vi "Read TCPClient.vi"(8 "error in (no error)":errorcluster, 11 "SpectrographClientCommunicator in":refnum<class "SpectrographClientCommunicator.lvclass">) -> (0 "error out":errorcluster, 2 "TCPClient":refnum<class "TCPClient.lvclass">, 3 "SpectrographClientCommunicator out":refnum<class "SpectrographClientCommunicator.lvclass">)   [LabVIEW 2016, in "SpectrographClientCommunicator.lvclass"]
uses:
  SpectrographClientCommunicator.lvclass
  ts_labview_tcp/TCPClient/TCPClient.lvclass
  SpectrographClientCommunicator.lvclass/SpectrographClientCommunicator.ctl
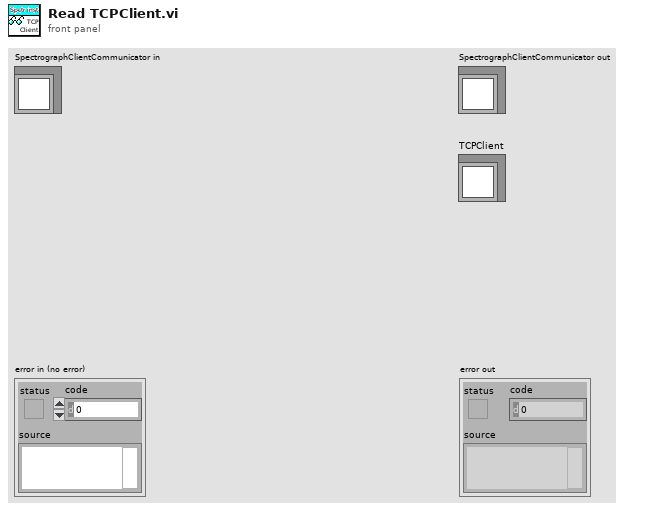
[diagram p1: front panel]
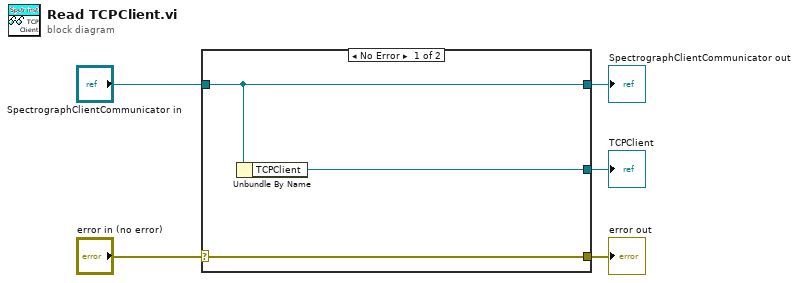
[diagram p0: block diagram]
diagram:
  n1 = case shown="No Error" "error in (no error)" {
    selector: "error in (no error)" -> [w8 w9]
    tunnel: [w8 w9] -> w4
    tunnel: [w7 w10] -> w2
    tunnel: "SpectrographClientCommunicator in" -> [w7 w10]
    tunnel: [w6 _] -> w1
    frame No Error {
      n2 = Unbundle By Name(w7) -> ("TCPClient"=w6:refnum<class "TCPClient.lvclass">)
    }
    frame Error {
    }
  }
  "error out" <- w4
  "SpectrographClientCommunicator out" <- w2
  "TCPClient" <- w1
